vi "Error Handler - Confirm Quit.vi"() -> (2 "exit confirmed":bool=TRUE, 3 "channel":T1)   [LabVIEW 2023, in "Message Queue Helper.lvlib"]
doc: "Queries the user to find out if the application should exit or not."
uses:
  <extravilib>/ChannelInstances/Messenger-t'Message Queue.lvlib-Message Cluster.ctl'/))Channel.ctl
  Message Cluster.ctl
  Enqueue Message.vi
  <extravilib>/ChannelInstances/Messenger-t'Message Queue.lvlib-Message Cluster.ctl'/Write.vi
  <extravilib>/ChannelInstances/Messenger-t'Message Queue.lvlib-Message Cluster.ctl'/Write With Abort.vi
  <extravilib>/ChannelInstances/Messenger-t'Message Queue.lvlib-Message Cluster.ctl'/Endpoint.vi
  Message Queue Helper.lvlib
  Message Queue.lvlib
  <extravilib>/ChannelInstances/Messenger-t'Message Queue.lvlib-Message Cluster.ctl'.lvlib
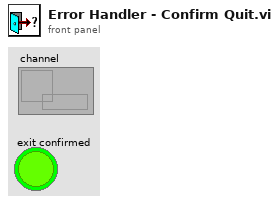
[diagram p1: front panel]
types:
  T1 = typedef "Messenger-t'Message Queue.lvlib-Message Cluster.ctl'.lvlib/))Channel.ctl" = refnum<queue>
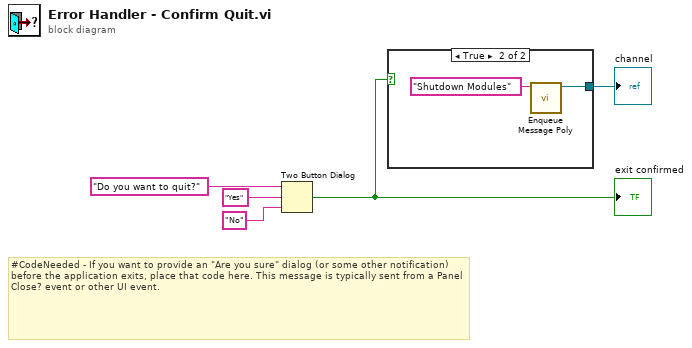
[diagram p0: block diagram]
diagram:
  # "#CodeNeeded - If you want to provide an \"Are you sure\" dialog (or some other notification) before the application exits, place that code here. This message is typically sent from a Panel Close? event or other UI event."
  n1 = Two Button Dialog(message="Do you want to quit?" ("Do you want to quit?"), 1:"No" ("No"), 2:"Yes" ("Yes")) -> (T button?=w4:bool)
  "exit confirmed" <- w4
  n2 = case shown="True" w4 {
    tunnel: [_ w7] -> w5
    frame False {
    }
    frame True {
      n3 = call-poly "Enqueue Message Poly.vi"("Message"="Shutdown Modules") -> ("channel"=w7:T1)  [unwired: 10 in]
    }
  }
  "channel" <- w5
